vi "DaqClose.vi"(8 "error in":errorcluster caption="错误输入", 11 "task in":refnum<k21> caption="任务输入") -> (0 "error out":errorcluster caption="错误输出")   [LabVIEW 2020]
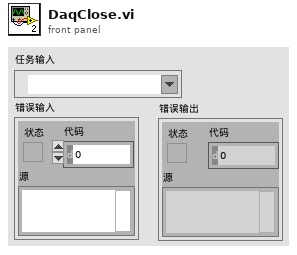
[diagram p1: front panel]
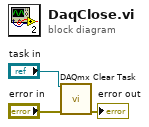
[diagram p0: block diagram]
diagram:
  n1 = call <vilib>:"DAQmx Clear Task.vi"("task in"="task in", "error in"="error in") -> ("error out"=→"error out":errorcluster)  [unwired: 13 in]
